vi "TableManager.vi"(6 "Fixed":T1={"FixedDays"=FALSE, "DaysBack"=7, "FixTrendDays"=FALSE, "DaysBackTrend"=0}, 8 "Op":T5(ring), 9 "PlotName":string, 10 "Level":u16(ring) items=["County", "State", "Country"], 11 "GeoData":T4) -> (1 "Strings":T2, 2 "FipsOut":i32[](array[numeric]), 3 "TableOut":string[][](table))   [LabVIEW 2017]
panel:
  out "Data":T3(array[cluster])
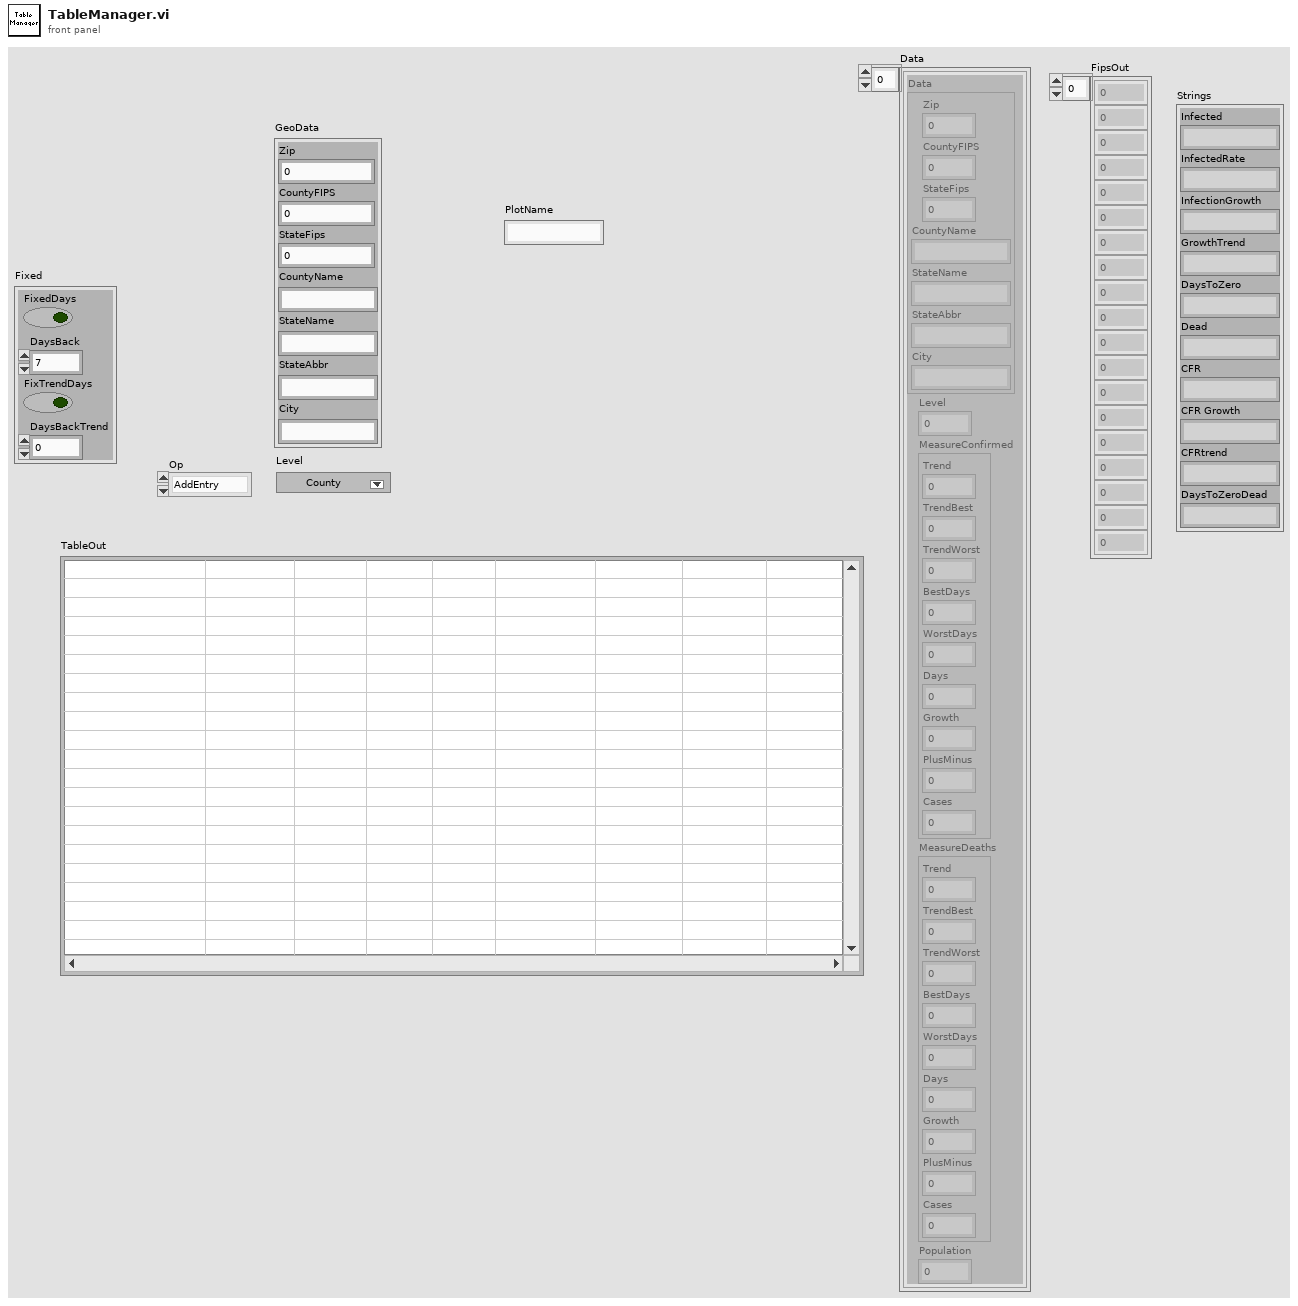
[diagram p1: front panel]
types:
  T1 = cluster{"FixedDays":bool, "DaysBack":i32, "FixTrendDays":bool, "DaysBackTrend":i32}
  T2 = cluster{"Infected":string, "InfectedRate":string, "InfectionGrowth":string, "GrowthTrend":string, "DaysToZero":string, "Dead":string, "CFR":string, "CFR Growth":string, "CFRtrend":string, "DaysToZeroDead":string}
  T3 = cluster{"Data":cluster{"Zip":i32, "CountyFIPS":i32, "StateFips":i32, "CountyName":string, "StateName":string, "StateAbbr":string, "City":string}, "Level":u16, "MeasureConfirmed":cluster{"Trend":dbl, "TrendBest":dbl, "TrendWorst":dbl, "BestDays":dbl, "WorstDays":dbl, "Days":dbl, "Growth":dbl, "PlusMinus":dbl, "Cases":i32}, "MeasureDeaths":cluster{"Trend":dbl, "TrendBest":dbl, "TrendWorst":dbl, "BestDays":dbl, "WorstDays":dbl, "Days":dbl, "Growth":dbl, "PlusMinus":dbl, "Cases":i32}, "Population":i32}[]
  T4 = cluster{"Zip":i32, "CountyFIPS":i32, "StateFips":i32, "CountyName":string, "StateName":string, "StateAbbr":string, "City":string}
  T5 = enum16{"AddEntry", "Clear", "Expand", "Combine", "GetStrings", "GetGeo"}
  T6 = cluster{"Data":cluster{"Zip":i32, "CountyFIPS":i32, "StateFips":i32, "CountyName":string, "StateName":string, "StateAbbr":string, "City":string}, "Level":u16, "MeasureConfirmed":cluster{"Trend":dbl, "TrendBest":dbl, "TrendWorst":dbl, "BestDays":dbl, "WorstDays":dbl, "Days":dbl, "Growth":dbl, "PlusMinus":dbl, "Cases":i32}, "MeasureDeaths":cluster{"Trend":dbl, "TrendBest":dbl, "TrendWorst":dbl, "BestDays":dbl, "WorstDays":dbl, "Days":dbl, "Growth":dbl, "PlusMinus":dbl, "Cases":i32}, "Population":i32}
  T7 = enum16{"LoadData", "GetStateData", "GetCountyData", "GetCountyArray"}
  T8 = enum16{"ClearCache", "AddPlot", "GetPlot", "GetNames"}
  T9 = cluster{"ConfirmedCases":i32[], "ConfirmedDeaths":i32[], "Days":timestamp[], "Population":i32}
  T10 = cluster{"ConfirmedCases":i32[], "Days":timestamp[]}
  T11 = cluster{"ConfirmedDeaths":i32[], "Days":timestamp[]}
  T12 = cluster{"Trend":dbl, "TrendBest":dbl, "TrendWorst":dbl, "BestDays":dbl, "WorstDays":dbl, "Days":dbl, "Growth":dbl, "PlusMinus":dbl, "Cases":i32}
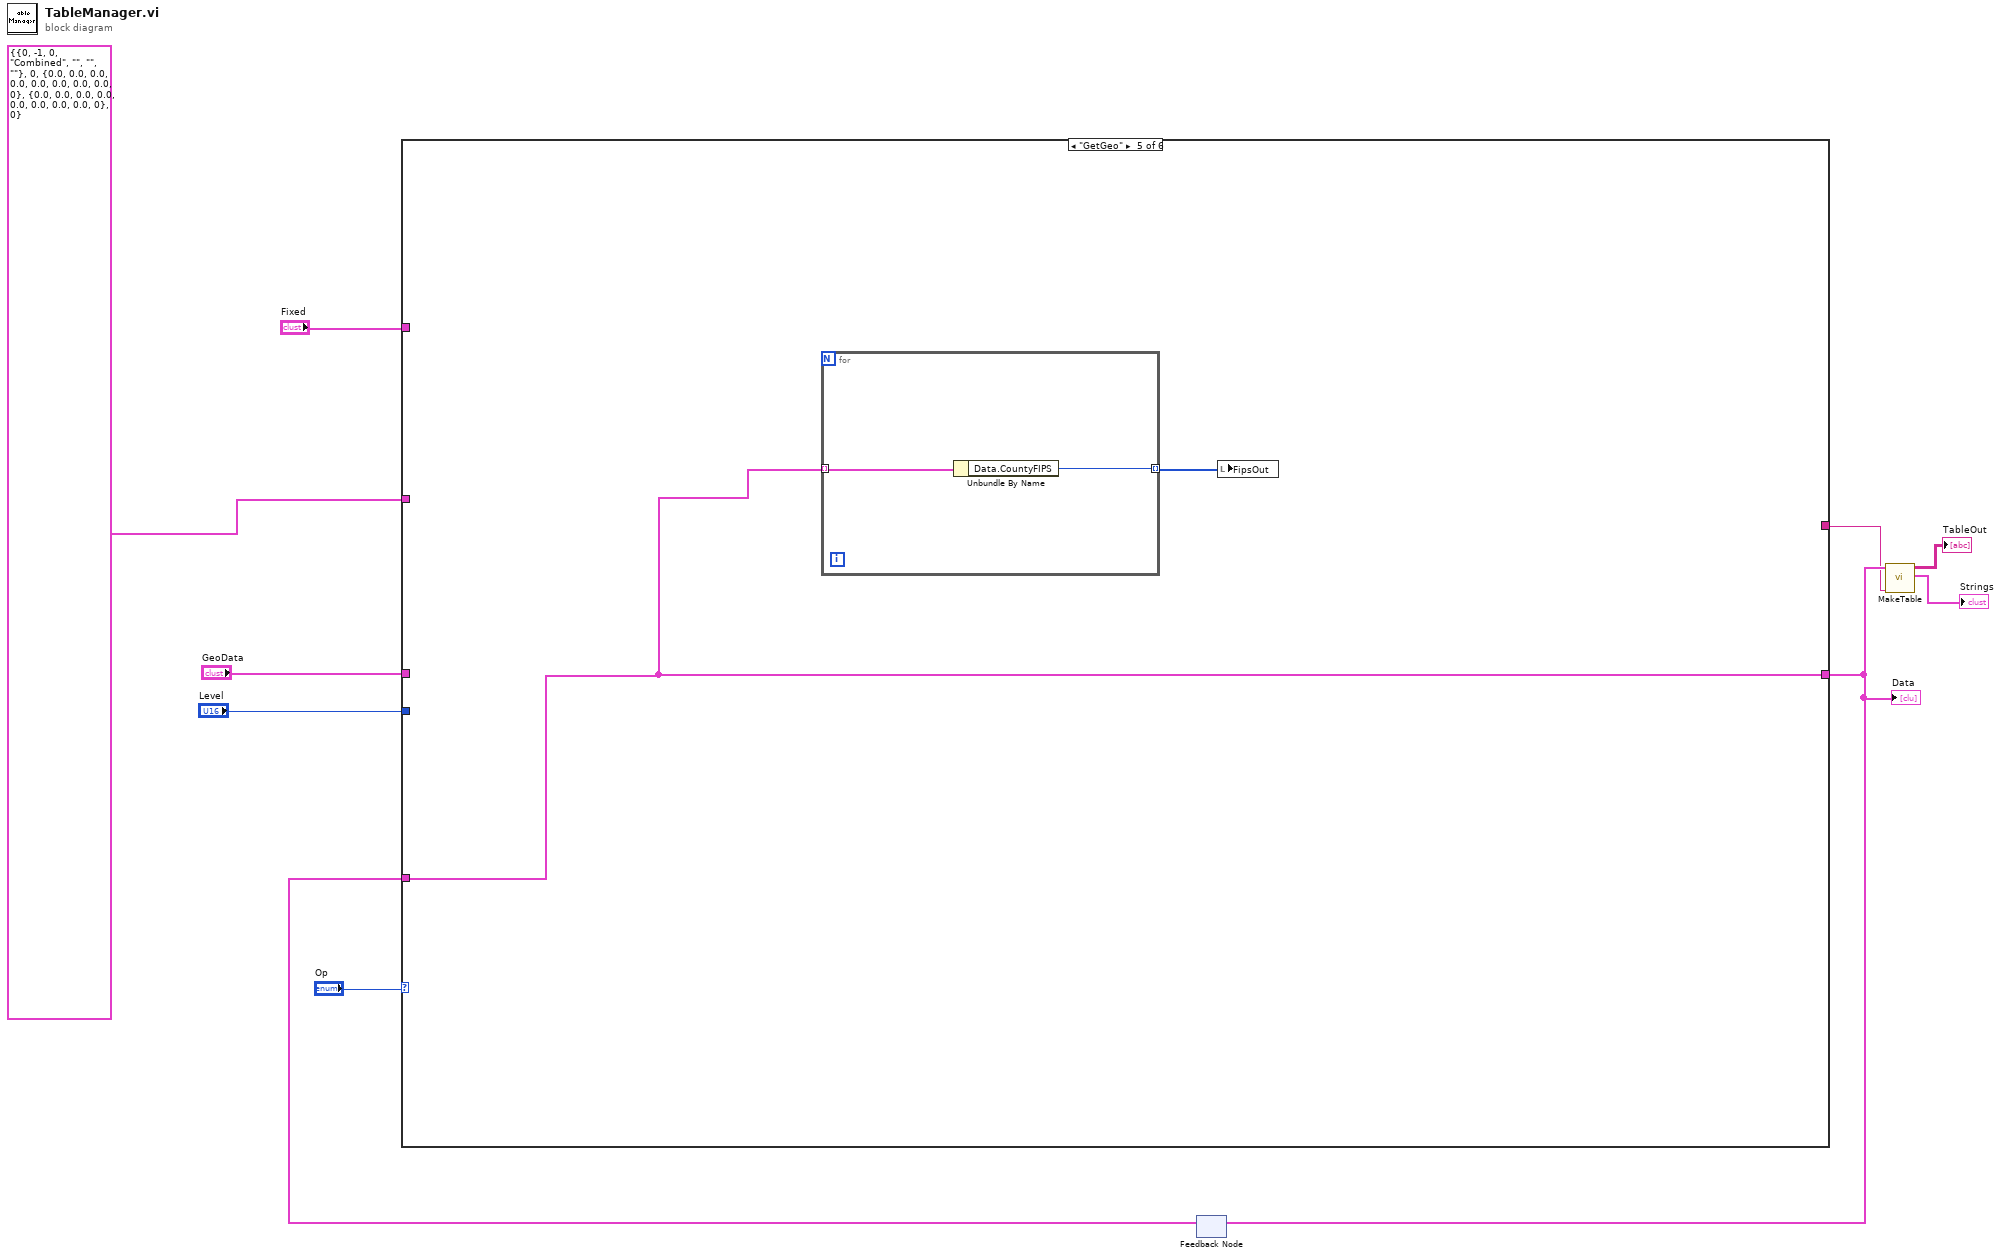
[diagram p0: block diagram]
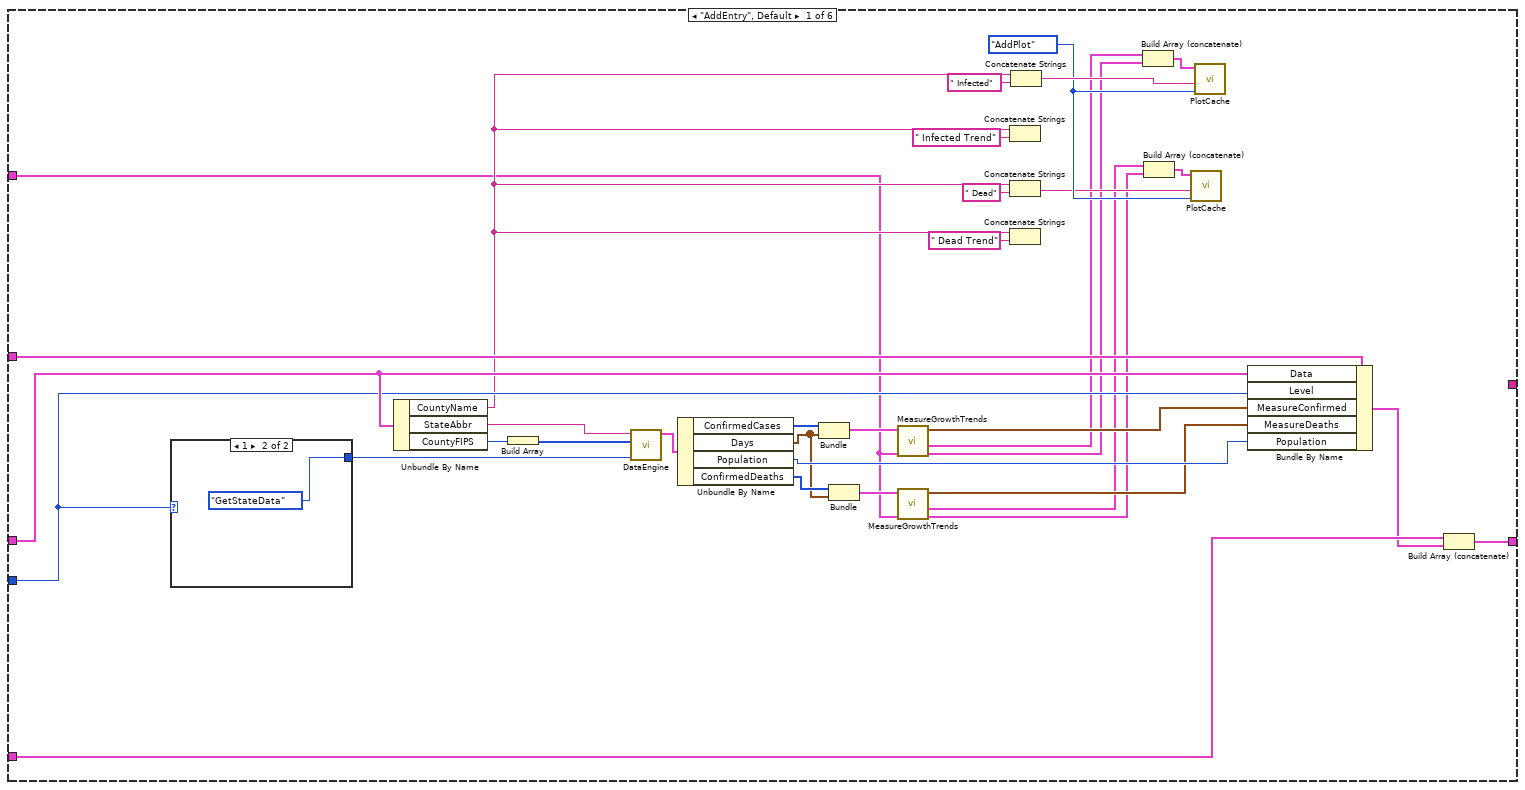
[diagram p2: hidden frame]
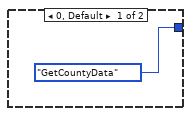
[diagram p3: hidden frame]
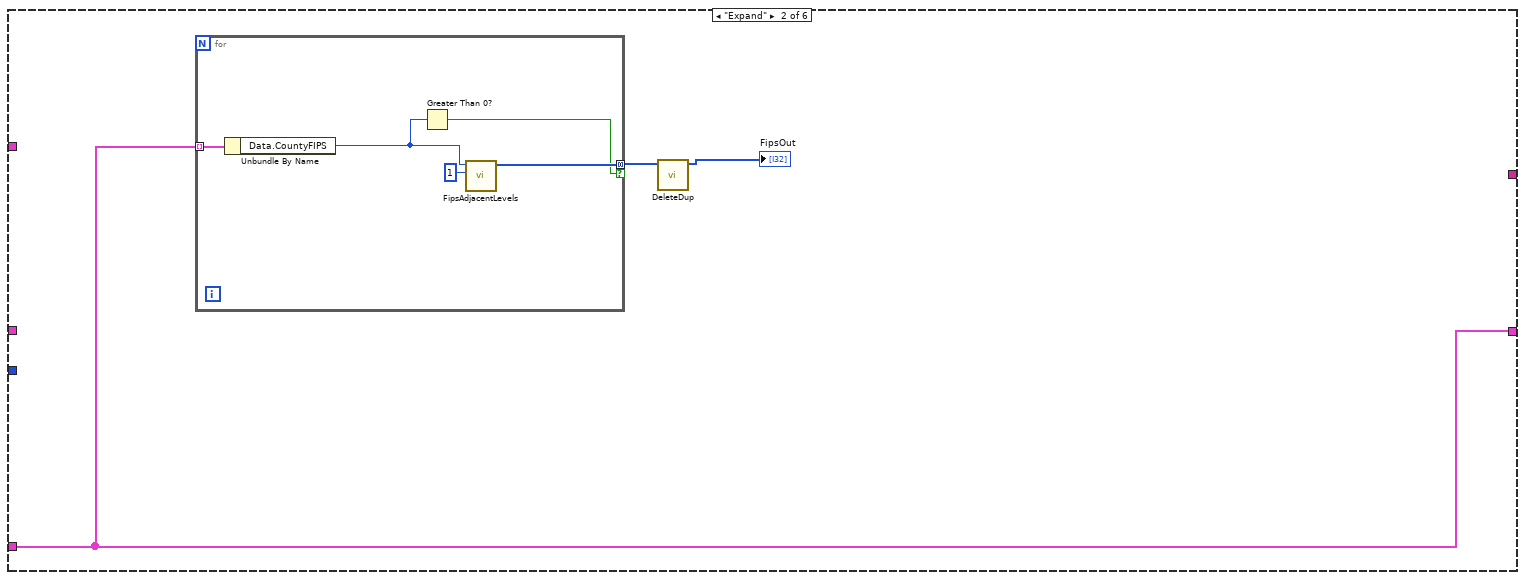
[diagram p4: hidden frame]
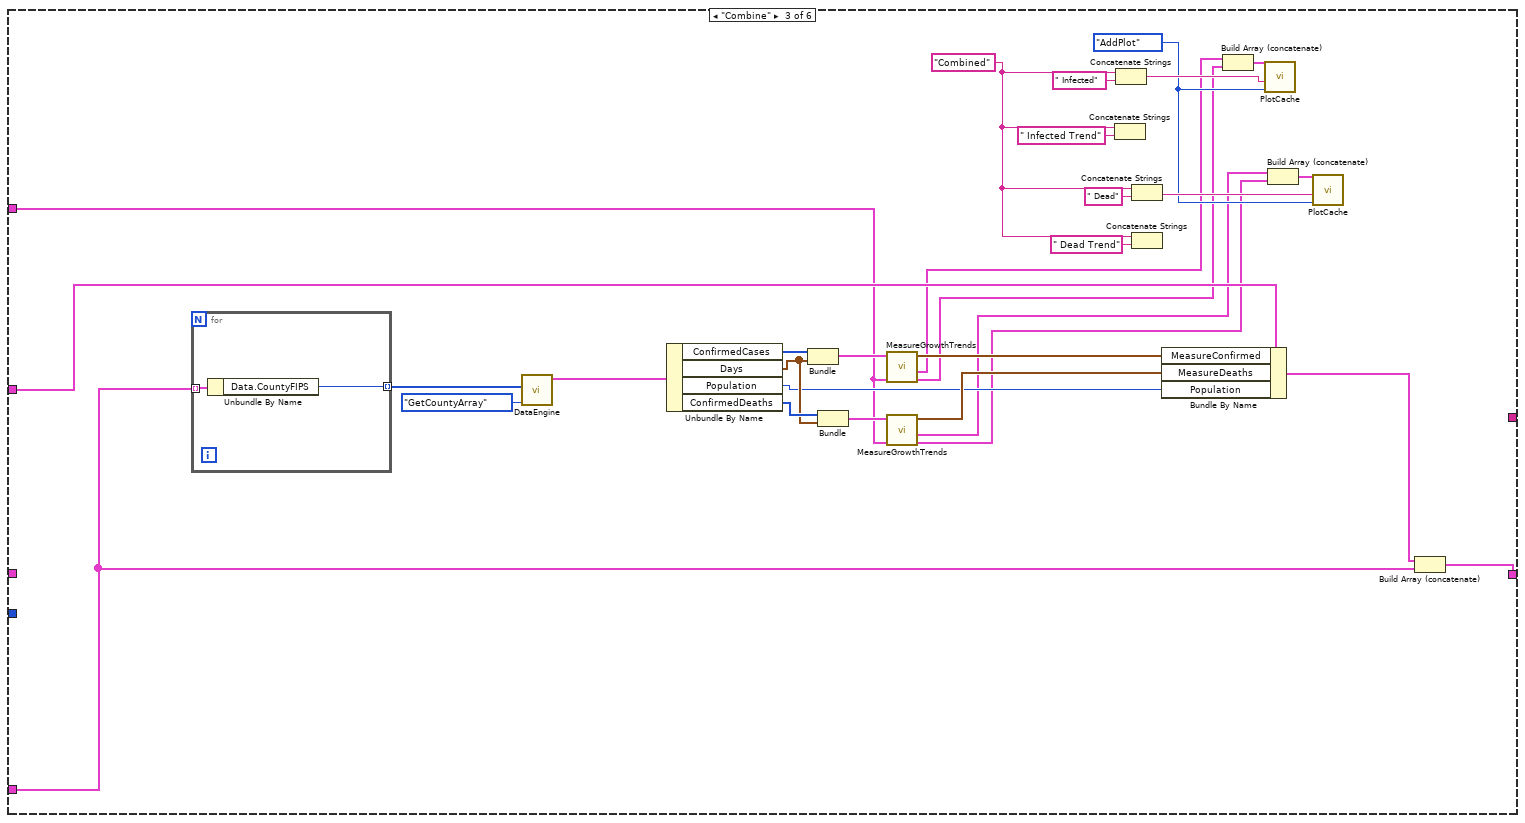
[diagram p5: hidden frame]
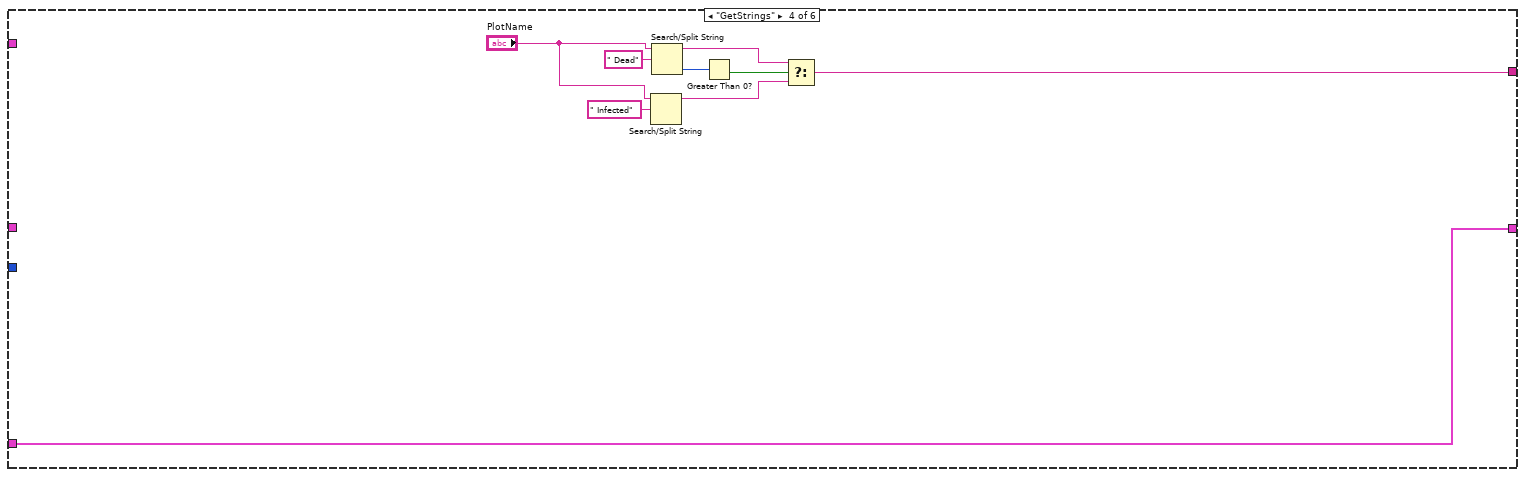
[diagram p6: hidden frame]
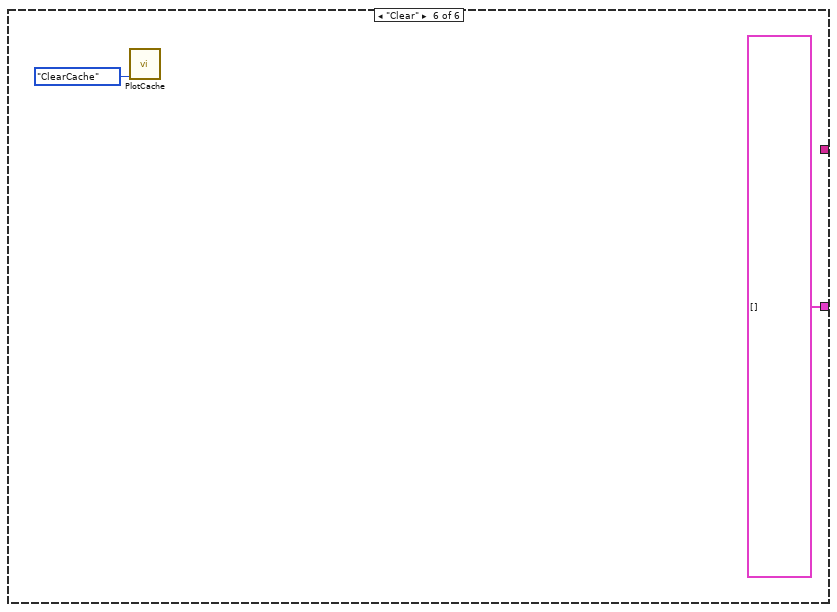
[diagram p7: hidden frame]
diagram:
  n1 = feedback #1() -> (w8:T3)  [unwired: 1 in]
  n2 = case shown="\"GetGeo\"" "Op" {
    tunnel: T6 {"Data"={"Zip"=0, "CountyFIPS"=-1, "StateFips"=0, "CountyName"="Combined", "StateName"="", "StateAbbr"="", "City"=""}, "Level"=0, "MeasureConfirmed"={"Trend"=0.0, "TrendBest"=0.0, "TrendWorst"=0.0, "BestDays"=0.0, "WorstDays"=0.0, "Days"=0.0, "Growth"=0.0, "PlusMinus"=0.0, "Cases"=0}, "MeasureDeaths"={"Trend"=0.0, "TrendBest"=0.0, "TrendWorst"=0.0, "BestDays"=0.0, "WorstDays"=0.0, "Days"=0.0, "Growth"=0.0, "PlusMinus"=0.0, "Cases"=0}, "Population"=0} -> [w44 _ w76 _ _ _]
    tunnel: w8 -> [w43 w49 w73 w95 w97 _]
    tunnel: [w42 w49 w72 w95 w97 T3 []] -> w5
    tunnel: "GeoData" -> [w41 _ _ _ _ _]
    tunnel: "Level" -> [w38 _ _ _ _ _]
    tunnel: [_ _ _ w87 _ _] -> w2
    tunnel: "Fixed" -> [w11 _ w55 _ _ _]
    frame "AddEntry", Default {
      w23 = T8."AddPlot" ("Op")
      n3 = case shown="1" w38 {
        tunnel: [T7."GetCountyData" ("Op") T7."GetStateData" ("Op")] -> w37
        frame 0, Default {
        }
        frame 1 {
        }
      }
      n4 = Unbundle By Name(w41) -> ("CountyName"=w19:string, "StateAbbr"=w36:string, "CountyFIPS"=w40:i32)
      n5 = Build Array(w40) -> (w39:i32[])
      n6 = call "DataEngine.vi"("Op"=w37, "Fips"=w39, "State"=w36) -> ("Data"=w35:T9)  [unwired: 7 in, 1 out]
      n7 = Unbundle By Name(w35) -> ("ConfirmedCases"=w34:i32[], "Days"=w29:timestamp[], "Population"=w31:i32, "ConfirmedDeaths"=w30:i32[])
      n8 = Bundle("ConfirmedCases"=w34, "Days"=w29) -> (w33:T10)  [unwired: 1 in]
      n9 = Bundle("ConfirmedDeaths"=w30, "Days"=w29) -> (w28:T11)  [unwired: 1 in]
      n10 = call "MeasureGrowthTrends.vi"("Fixed"=w11, "Data"=w33) -> ("Trend"=w16:cluster{"Days":timestamp[], dbl[]}[], "Growth"=w17:cluster{"Days":timestamp[], dbl[]}[], "Measure"=w32:T12)  [unwired: 7 in]
      n11 = call "MeasureGrowthTrends.vi"("Fixed"=w11, "Data"=w28) -> ("Trend"=w13:cluster{"Days":timestamp[], dbl[]}[], "Growth"=w14:cluster{"Days":timestamp[], dbl[]}[], "Measure"=w27:T12)  [unwired: 7 in]
      n12 = Concatenate Strings(w19, " Infected Trend" ("string")) -> ()  [unwired: 1 out]
      n13 = Concatenate Strings(w19, " Dead" ("string")) -> (w18:string)
      n14 = Concatenate Strings(w19, " Dead Trend" ("string")) -> ()  [unwired: 1 out]
      n15 = Concatenate Strings(w19, " Infected" ("string")) -> (w24:string)
      n16 = Build Array (concatenate)(w17, w16) -> (w15:cluster{"Days":timestamp[], dbl[]}[])
      n17 = Build Array (concatenate)(w14, w13) -> (w12:cluster{"Days":timestamp[], dbl[]}[])
      n18 = call "PlotCache.vi"("Op"=w23, "PlotName"=w18, "Plot"=w12) -> ()  [unwired: 6 in, 3 out]
      n19 = call "PlotCache.vi"("Op"=w23, "PlotName"=w24, "Plot"=w15) -> ()  [unwired: 6 in, 3 out]
      n20 = Bundle By Name(cluster=w44, "Data"=w41, "Level"=w38, "MeasureConfirmed"=w32, "MeasureDeaths"=w27, "Population"=w31) -> (w26:T6)
      n21 = Build Array (concatenate)(w43, w26) -> (w42:T3)
    }
    frame "Expand" {
      n22 = for {
        tunnel: [w53] -> w48 mode=concatenating if=w50
        tunnel: w49 -> [w52] mode=indexing
        n23 = Unbundle By Name(w52) -> ("Data.CountyFIPS"=w51:i32)
        n24 = Greater Than 0?(x=w51) -> (x > 0?=w50:bool)
        n25 = call "FipsAdjacentLevels.vi"("Levels"=1, "Fips"=w51) -> ("FipsOut"=w53:i32[])  [unwired: 9 in]
      }
      n26 = call "DeleteDup.vi"("Array in"=w48) -> ("Array out"=→"FipsOut":i32[])  [unwired: 10 in]
    }
    frame "Combine" {
      w63 = "Combined" ("string")
      w62 = T8."AddPlot" ("Op")
      n27 = for {
        tunnel: w73 -> [w86] mode=indexing
        tunnel: [w85] -> w84 mode=indexing
        n28 = Unbundle By Name(w86) -> ("Data.CountyFIPS"=w85:i32)
      }
      n29 = call "DataEngine.vi"("Op"=T7."GetCountyArray", "Fips"=w84) -> ("Data"=w77:T9)  [unwired: 8 in, 1 out]
      n30 = Unbundle By Name(w77) -> ("ConfirmedCases"=w82:i32[], "Days"=w79:timestamp[], "Population"=w71:i32, "ConfirmedDeaths"=w80:i32[])
      n31 = Bundle("ConfirmedCases"=w82, "Days"=w79) -> (w81:T10)  [unwired: 1 in]
      n32 = Bundle("ConfirmedDeaths"=w80, "Days"=w79) -> (w78:T11)  [unwired: 1 in]
      n33 = call "MeasureGrowthTrends.vi"("Fixed"=w55, "Data"=w81) -> ("Trend"=w60:cluster{"Days":timestamp[], dbl[]}[], "Growth"=w61:cluster{"Days":timestamp[], dbl[]}[], "Measure"=w75:T12)  [unwired: 7 in]
      n34 = call "MeasureGrowthTrends.vi"("Fixed"=w55, "Data"=w78) -> ("Trend"=w57:cluster{"Days":timestamp[], dbl[]}[], "Growth"=w58:cluster{"Days":timestamp[], dbl[]}[], "Measure"=w74:T12)  [unwired: 7 in]
      n35 = Concatenate Strings(w63, " Infected Trend" ("string")) -> ()  [unwired: 1 out]
      n36 = Concatenate Strings(w63, " Infected" ("string")) -> (w68:string)
      n37 = Concatenate Strings(w63, " Dead" ("string")) -> (w64:string)
      n38 = Concatenate Strings(w63, " Dead Trend" ("string")) -> ()  [unwired: 1 out]
      n39 = Bundle By Name(cluster=w76, "MeasureConfirmed"=w75, "MeasureDeaths"=w74, "Population"=w71) -> (w70:T6)
      n40 = Build Array (concatenate)(w61, w60) -> (w59:cluster{"Days":timestamp[], dbl[]}[])
      n41 = call "PlotCache.vi"("Op"=w62, "PlotName"=w68, "Plot"=w59) -> ()  [unwired: 6 in, 3 out]
      n42 = Build Array (concatenate)(w58, w57) -> (w56:cluster{"Days":timestamp[], dbl[]}[])
      n43 = call "PlotCache.vi"("Op"=w62, "PlotName"=w64, "Plot"=w56) -> ()  [unwired: 6 in, 3 out]
      n44 = Build Array (concatenate)(w70, w73) -> (w72:T3)
    }
    frame "GetStrings" {
      n45 = Search/Split String(string="PlotName", search string/char (-)=" Infected") -> (substring before match=w88:string)  [unwired: 1 in, 2 out]
      n46 = Search/Split String(string="PlotName", search string/char (-)=" Dead") -> (substring before match=w89:string, offset of match=w93:i32)  [unwired: 1 in, 1 out]
      n47 = Greater Than 0?(x=w93) -> (x > 0?=w90:bool)
      n48 = Select(t=w89, s=w90, f=w88) -> (s? t:f=w87:string)
    }
    frame "GetGeo" {
      n49 = for {
        tunnel: w97 -> [w99] mode=indexing
        tunnel: [w98] -> w96 mode=indexing
        n50 = Unbundle By Name(w99) -> ("Data.CountyFIPS"=w98:i32)
      }
      n51 = local write "FipsOut"(w96) -> ()
    }
    frame "Clear" {
      n52 = call "PlotCache.vi"("Op"=T8."ClearCache") -> ()  [unwired: 8 in, 3 out]
    }
  }
  "Data" <- w5
  n53 = feedback-in #1(w5) -> ()
  n54 = call "MakeTable.vi"("PlotCounty"=w2, "TableData"=w5) -> ("Strings"=→"Strings":T2, "TableOut"=→"TableOut":string[][])  [unwired: 8 in]
